vi "BuildServerTitleText.vi"(3 "ROS":T1) -> (0 "text":string, 1 "colored text":string)   [LabVIEW 2012]
uses:
  <userlib>/ROSforLV/ROS/Code/SubVIs/_ROSControl.ctl
  <userlib>/ROSforLV/ROS/Code/SubVIs/_ROSDirection.ctl
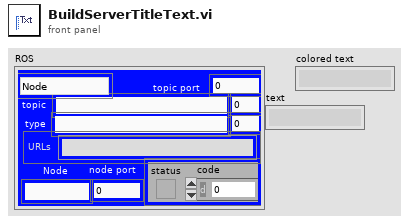
[diagram p1: front panel]
types:
  T1 = typedef "_ROSControl.ctl" = cluster{"topic port":u16, "Node":string, "topic":string, "type":string, "node port":u32, "error ":errorcluster, "Direction":T2, "APIs":string[], "Update (ms)":u16, "write queue":u16}
  T2 = typedef "_ROSDirection.ctl" = enum16{"Node", "Publisher", "Subscriber", "Service Client"}
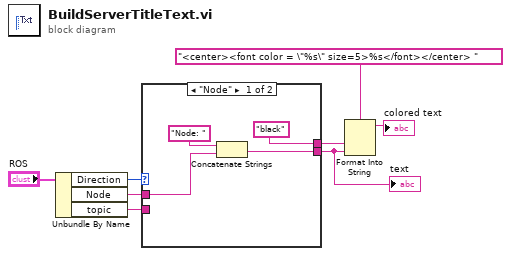
[diagram p0: block diagram]
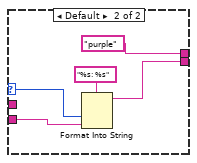
[diagram p2: hidden frame]
diagram:
  n1 = Unbundle By Name("ROS") -> ("Direction"=w5:T2, "Node"=w6:string, "topic"=w7:string)
  n2 = case shown="\"Node\"" w5 {
    selector: w5 -> [_ w16]
    tunnel: w6 -> [w10 _]
    tunnel: w7 -> [_ w15]
    tunnel: [w9 w14] -> w1
    tunnel: ["black" ("format string") "purple" ("format string")] -> w3
    frame "Node" {
      n3 = Concatenate Strings("Node: " ("format string"), w10) -> (w9:string)
    }
    frame Default {
      n4 = Format Into String(format string="%s: %s", w16, w15) -> (resulting string=w14:string)  [unwired: 2 in, 1 out]
    }
  }
  "text" <- w1
  n5 = Format Into String(format string="<center><font color = \"%s\" size=5>%s</font></center> " ("string"), w3, w1) -> (resulting string=→"colored text":string)  [unwired: 2 in, 1 out]
